vi "BioFeedback2(AudioInput+FirstFilteringAttempt).vi"() -> ()   [LabVIEW 2016]
uses:
  <vilib>/Analysis/5stat.llb/RMS (DBL).vi
  <vilib>/Analysis/baseanly.llb/Mean (DBL).vi
  <vilib>/Analysis/NI_AALBase.lvlib
  <vilib>/Analysis/NI_AALPro.lvlib
panel:
  in  "sample duration":dbl
  out "RMS 2":waveform(dbl)(graph)
  out "filetered RMS Value 2":dbl
  out "RMS":waveform(dbl)(graph)
  out "RMS Value":dbl
  out "filtered":waveform(dbl)(graph)
  out "filtered + positivepeaks":waveform(dbl)(graph)
  out "Peaks Waveform (OLD)":waveform(dbl)(graph)
  out "Raw Audio\nWaveform":waveform(dbl)(graph)
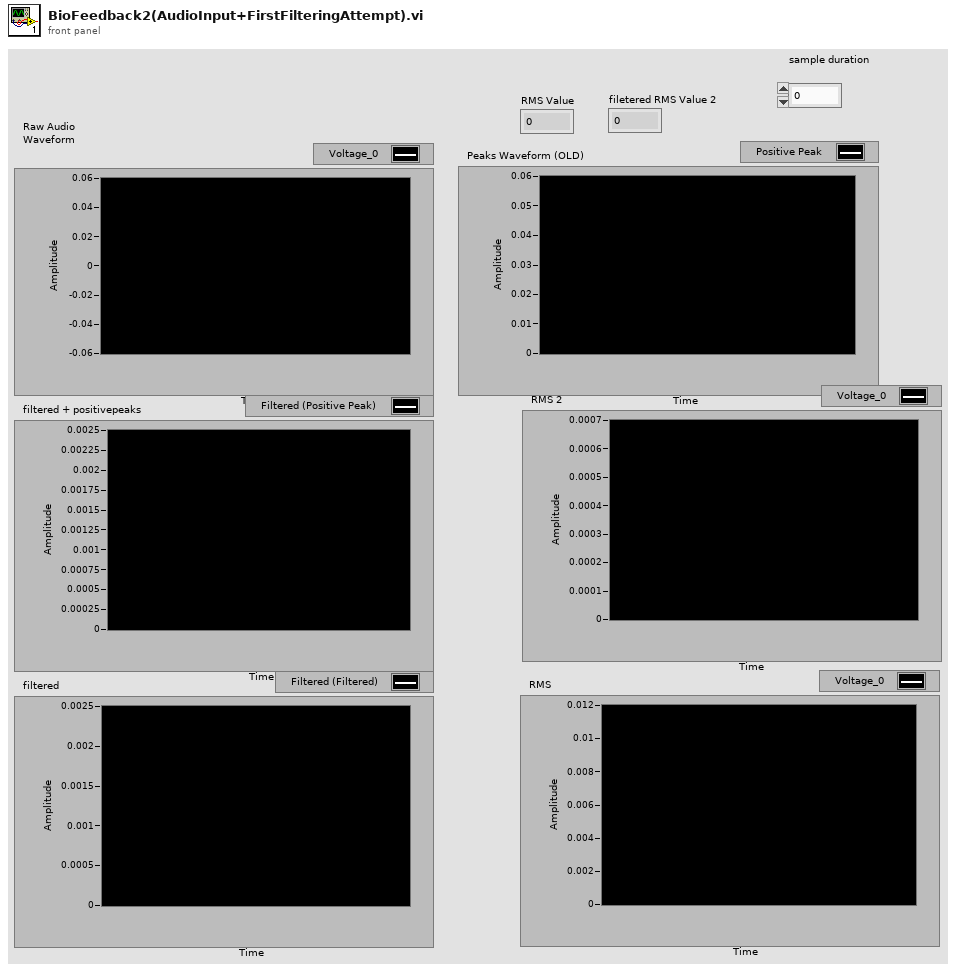
[diagram p1: front panel]
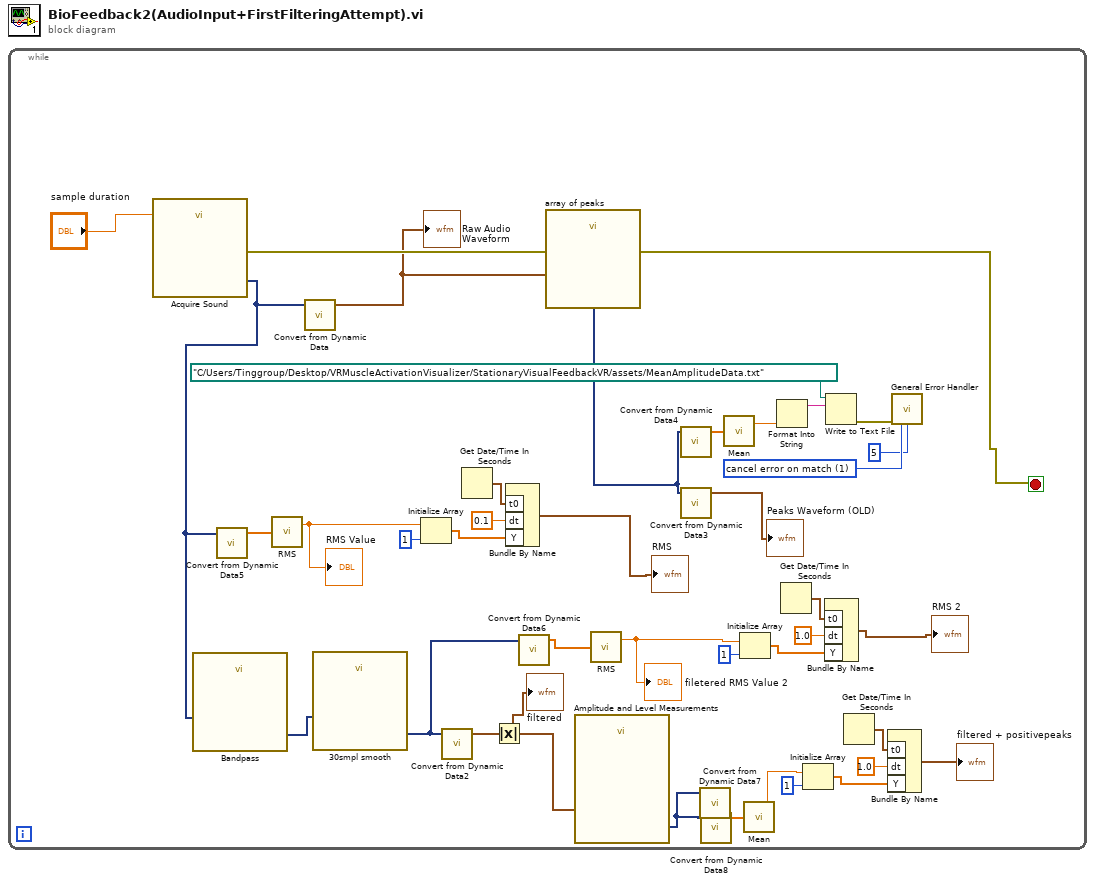
[diagram p0: block diagram]
diagram:
  n1 = while {
    stop <- w34 stop-if-true
    w38 = 1 items=["no exception", "cancel error on match", "set error on match"] ("[exception action] (none:0)")
    n2 = call "Acquire Sound"("Duration (s)"="sample duration") -> ("Data"=w28:dynamicdata, "error out"=w34:errorcluster)  [unwired: 17 in]
    n3 = call "Bandpass"("Signal"=w28) -> ("Filtered Signal"=w29:dynamicdata)  [unwired: 9 in, 1 out]
    n4 = call "Convert from Dynamic Data5"("Dynamic Data Type"=w28) -> ("Array"=w27:dbl[])  [unwired: 3 in]
    n5 = call-poly <vilib>:"RMS.vi"("X"=w27) -> ("rms value"=w13:dbl)  [unwired: 1 out]
    "RMS Value" <- w13
    n6 = call "Convert from Dynamic Data"("Dynamic Data Type"=w28, "Channel"=w28) -> ("Waveform"=w32:waveform(dbl))  [unwired: 2 in]
    "Raw Audio\nWaveform" <- w32
    n7 = call "30smpl smooth"("Signal"=w29) -> ("Filtered Signal"=w17:dynamicdata)  [unwired: 9 in, 1 out]
    n8 = Initialize Array(w13, 1 ("dimension size")) -> (w25:dbl[])
    n9 = call "Convert from Dynamic Data2"("Dynamic Data Type"=w17) -> ("Waveform"=w18:waveform(dbl))  [unwired: 3 in]
    n10 = Get Date/Time In Seconds() -> (seconds since 1Jan1904=w31:timestamp)
    n11 = Absolute Value(x=w18) -> (abs(x)=w14:waveform(dbl))
    "filtered" <- w14
    n12 = Bundle By Name("t0"=w31, "dt"=0.1, "Y"=w25) -> (→"RMS":waveform(dbl))  [unwired: 1 in]
    n13 = call "Convert from Dynamic Data6"("Dynamic Data Type"=w17) -> ("Array"=w16:dbl[])  [unwired: 3 in]
    n14 = call "array of peaks"("Signals"=w32) -> ("Positive Peak"=w33:dynamicdata)  [unwired: 13 in, 1 out]
    n15 = call "Amplitude and Level Measurements"("Signals"=w14) -> ("Positive Peak"=w10:dynamicdata)  [unwired: 13 in, 1 out]
    n16 = call-poly <vilib>:"RMS.vi"("X"=w16) -> ("rms value"=w21:dbl)  [unwired: 1 out]
    "filetered RMS Value 2" <- w21
    n17 = call "Convert from Dynamic Data4"("Dynamic Data Type"=w33) -> ("Array"=w12:dbl[])  [unwired: 3 in]
    n18 = call "Convert from Dynamic Data3"("Dynamic Data Type"=w33) -> ("Waveform"=→"Peaks Waveform (OLD)":waveform(dbl))  [unwired: 3 in]
    n19 = call "Convert from Dynamic Data7"("Dynamic Data Type"=w10) -> ()  [unwired: 3 in, 1 out]
    n20 = call "Convert from Dynamic Data8"("Dynamic Data Type"=w10) -> ("Array"=w11:dbl[])  [unwired: 3 in]
    n21 = call-poly <vilib>:"Mean.vi"("X"=w12) -> ("mean"=w3:dbl)  [unwired: 1 out]
    n22 = Initialize Array(w21, 1 ("dimension size")) -> (w19:dbl[])
    n23 = call-poly <vilib>:"Mean.vi"("X"=w11) -> ("mean"=w5:dbl)  [unwired: 1 out]
    n24 = Format Into String(w3) -> (resulting string=w36:string)  [unwired: 3 in, 1 out]
    n25 = Get Date/Time In Seconds() -> (seconds since 1Jan1904=w23:timestamp)
    n26 = Initialize Array(w5, 1 ("dimension size")) -> (w4:dbl[])
    n27 = Bundle By Name("t0"=w23, "dt"=1.0, "Y"=w19) -> (→"RMS 2":waveform(dbl))  [unwired: 1 in]
    n28 = Write to Text File(file (use dialog)=path "C:/Users/Tinggroup/Desktop/VRMuscleActivationVisualizer/StationaryVisualFeedbackVR/assets/MeanAmplitudeData.txt", text=w36) -> (error out=w39:errorcluster)  [unwired: 2 in, 2 out]
    n29 = Get Date/Time In Seconds() -> (seconds since 1Jan1904=w9:timestamp)
    n30 = Bundle By Name("t0"=w9, "dt"=1.0, "Y"=w4) -> (→"filtered + positivepeaks":waveform(dbl))  [unwired: 1 in]
    n31 = call <vilib>:"General Error Handler.vi"("error in (no error)"=w39, "[exception action] (none:0)"=w38, "[exception code]"=5) -> ()  [unwired: 8 in, 5 out]
  }
